vi "Store Configuration Parameters.vi"(8 "error in (no error)":errorcluster, 10 "refnum":T1, 11 "Example Configuration Dialog in":refnum<class "MotionSystem Configuration.lvclass">) -> (0 "error out":errorcluster, 2 "refnum out":T1, 3 "Example Configuration Dialog out":refnum<class "MotionSystem Configuration.lvclass">)   [LabVIEW 2016, in "MotionSystem.lvlib" / "MotionSystem Configuration.lvclass"]
uses:
  <userlib>/Common Components/Hardware/Abstract System/MotionSystem/MotionSystem Config/MotionSystem Configuration.lvclass
  <vilib>/Utility/config.llb/Config Data RefNum.ctl
  <userlib>/Common Components/Hardware/Abstract System/MotionSystem/MotionSystem Config/SectionName-MotionSystem.ctl
  <userlib>/Common Components/Hardware/Abstract System/MotionSystem/MotionSystem Config/MotionSystem Configuration.lvclass/MotionSystem Configuration.ctl
  <userlib>/Common Components/Hardware/Motor/Motor Config/Motor Configuration.lvclass
  <userlib>/Common Components/Hardware/Motor/Motor Config/Accessors/Write Motor Obj.vi
  <userlib>/Configuration Dialog Actor/Configuration.lvclass
  <userlib>/Common Components/Hardware/Abstract System/MotionSystem/MotionSystem/MotionSystem.lvclass
  <vilib>/Utility/config.llb/NI_LVConfig.lvlib
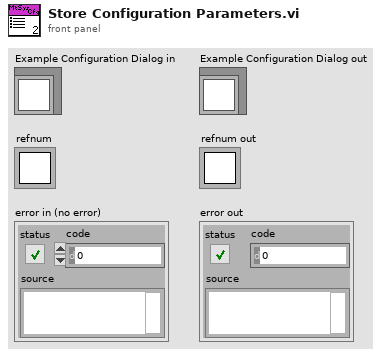
[diagram p1: front panel]
types:
  T1 = typedef "NI_LVConfig.lvlib/Config Data RefNum.ctl" = refnum<k1>
  T2 = typedef "MotionSystem.lvlib/MotionSystem Configuration.lvclass/SectionName-MotionSystem.ctl" = string
  T3 = typedef "MotionSystem.lvlib/MotionSystem Configuration.lvclass/RxRyZ Limits.ctl" = cluster{"Rx (deg)":cluster{"label":string, "soft limit min":dbl, "soft limit max":dbl}, "Ry (deg)":cluster{"label":string, "soft limit min":dbl, "soft limit max":dbl}, "Z (um)":cluster{"label":string, "soft limit min":dbl, "soft limit max":dbl}}
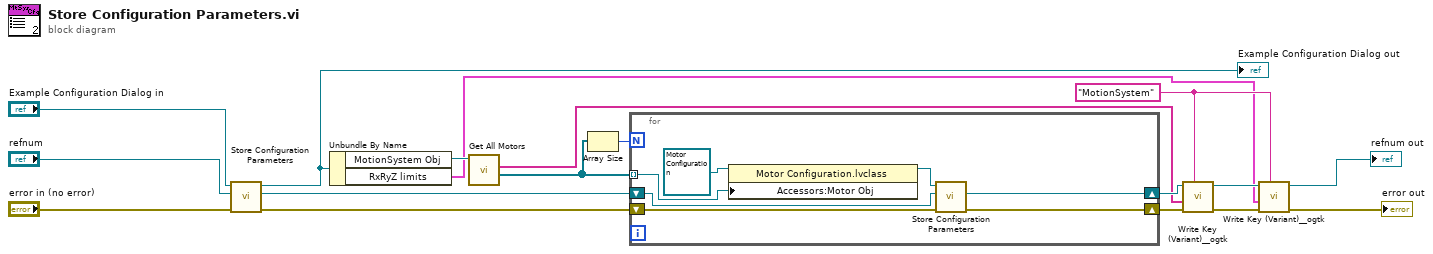
[diagram p0: block diagram]
diagram:
  w2 = T2 "MotionSystem" ("String")
  n1 = call-parent "Store Configuration Parameters.vi"("error in (no error)"="error in (no error)", "refnum"="refnum", "Configuration in"="Example Configuration Dialog in") -> ("error out"=w13:errorcluster, "refnum out"=w14:T1, "Configuration out"=w15:refnum<class "MotionSystem Configuration.lvclass">)  [unwired: 6 in]
  "Example Configuration Dialog out" <- w15
  n2 = Unbundle By Name(w15) -> ("MotionSystem Obj"=w9:refnum<class "MotionSystem.lvclass">, "RxRyZ limits"=w1:T3)
  n3 = call <userlib>:"Get All Motors.vi"("MotionSystem in"=w9) -> ("motors"=w7:refnum<class "Motor.lvclass">[], "labels"=w6:string[])  [unwired: 7 in, 2 out]
  n4 = Array Size(array=w7) -> (size(s)=w8:i32)
  n5 = for {
    N: w8 -> [_]
    shift-right: [w23] -> w10
    shift-left: w14 -> [w25]
    shift-right: [w22] -> w12
    shift-left: w13 -> [w24]
    tunnel: w7 -> [w20] mode=indexing
    n6 = property class="Motor Configuration.lvclass"(reference=refnum<class "Motor Configuration.lvclass"> refnum ("Hardware.lvlib:Motor.lvlib:Motor Configuration.lvclass"), "Accessors:Motor Obj"=w20) -> (reference out=w19:refnum<class "Motor Configuration.lvclass">)  [unwired: 1 in, 1 out]
    n7 = call-dynamic "Store Configuration Parameters.vi"("error in (no error)"=w24, "refnum"=w25, "Example Configuration Dialog in"=w19) -> ("error out"=w22:errorcluster, "refnum out"=w23:T1)  [unwired: 6 in, 1 out]
  }
  n8 = call <userlib>:"Write Key (Variant)__ogtk.vi"("section"=w2, "error in (no error)"=w12, "key-value"=w6, "refnum"=w10) -> ("error out"=w11:errorcluster, "refnum out"=w4:T1)  [unwired: 6 in]
  n9 = call <userlib>:"Write Key (Variant)__ogtk.vi"("section"=w2, "error in (no error)"=w11, "key-value"=w1, "refnum"=w4) -> ("error out"=→"error out":errorcluster, "refnum out"=→"refnum out":T1)  [unwired: 6 in]
